vi "LV2013 eZAuto Detect Arduino.vi"(8 "error in (no error)":errorcluster) -> (0 "error out":errorcluster, 2 "Board Type (Uno)":T1, 3 "VISA resource name":refnum<visa-resource-name>)   [LabVIEW 2013]
doc: "Based on the original LIFA base, It returns the Board type as well"
uses:
  <vilib>/LabVIEW Interface for Arduino/Type Defs/Board Type.ctl
  <vilib>/LabVIEW Interface for Arduino/LabVIEW Interface for Arduino.lvlib
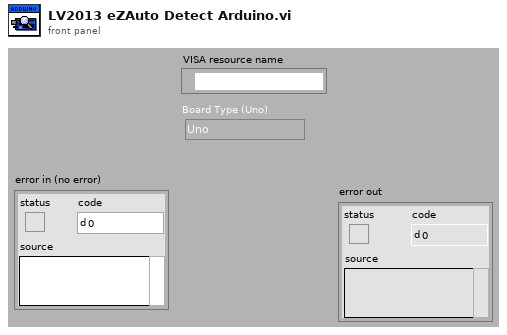
[diagram p1: front panel]
types:
  T1 = typedef "LabVIEW Interface for Arduino.lvlib/Board Type.ctl" = enum16{"Uno", "Dimuelanove w/Atmega 328", "Mega 2560"}
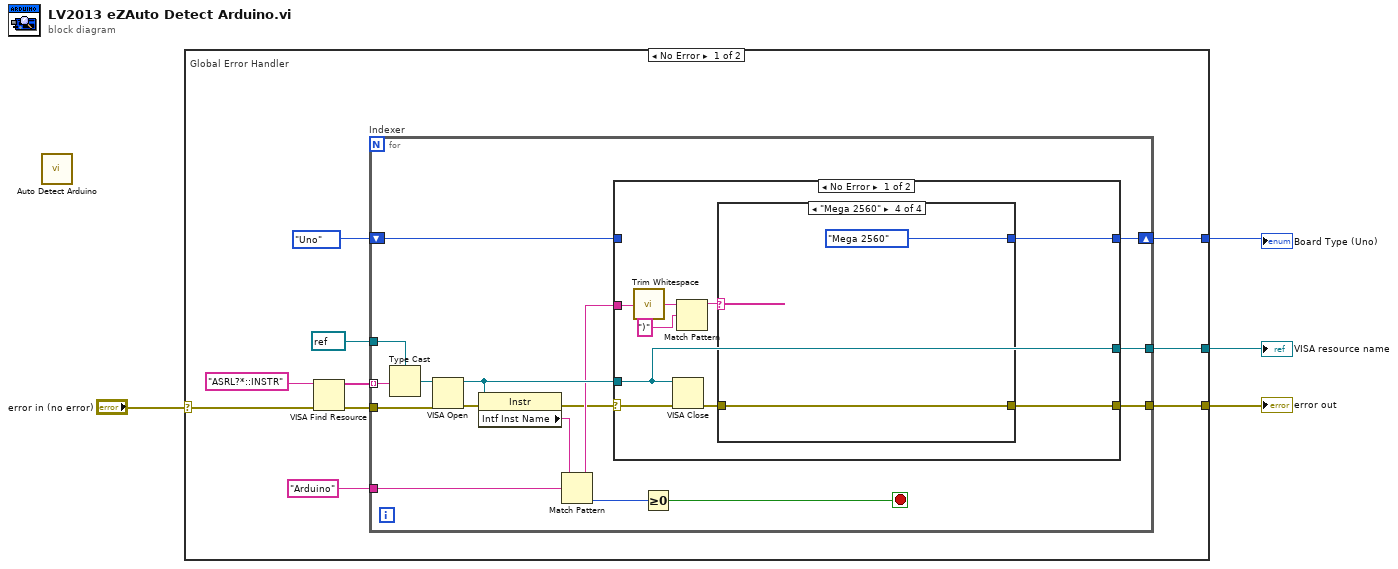
[diagram p0: block diagram]
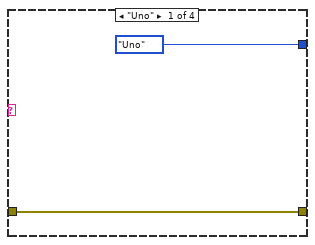
[diagram p2: hidden frame]
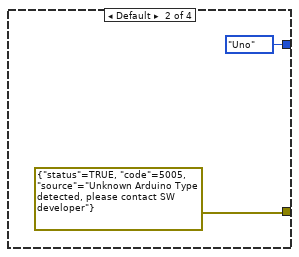
[diagram p3: hidden frame]
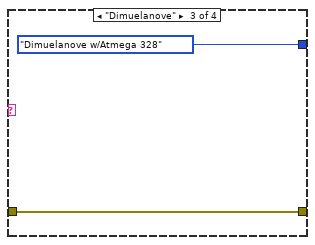
[diagram p4: hidden frame]
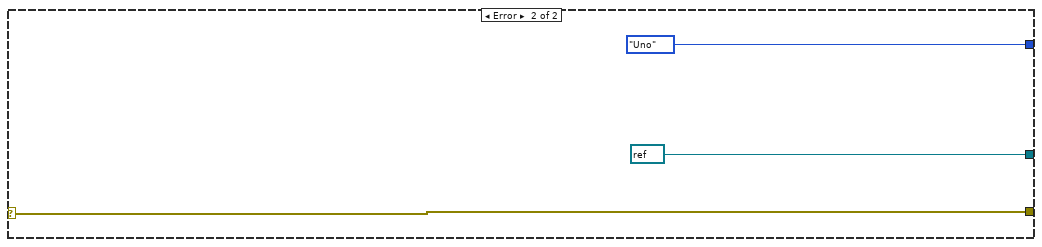
[diagram p6: hidden frame]
diagram:
  n1 = call <vilib>:"Auto Detect Arduino.vi"() -> ()  [unwired: 14 in, 2 out]
  n2 = case "Global Error Handler" shown="No Error" "error in (no error)" {
    selector: "error in (no error)" -> [w9 w51]
    tunnel: [w7 refnum<visa-resource-name> refnum ("VISA resource name")] -> w3
    tunnel: [w10 Board_Type."Uno" ("Board Type (Uno)")] -> w2
    tunnel: [w6 w51] -> w1
    frame No Error {
      n3 = VISA Find Resource(8:w9, 11:"ASRL?*::INSTR" ("expression (\"\")")) -> (0:w8:errorcluster, 3:w13:string[])  [unwired: 1 in, 1 out]
      n4 = for "Indexer" {
        tunnel: w13 -> [w29] mode=indexing
        tunnel: refnum<visa-resource-name> refnum ("VISA resource name") -> [w30]
        shift-right: [w26] -> w10
        shift-left: Board_Type."Uno" ("Board Type (Uno)") -> [w27]
        tunnel: w8 -> [w25]
        tunnel: [w17] -> w7
        tunnel: [w16] -> w6
        tunnel: "Arduino" -> [w15]
        stop <- w18 stop-if-true
        n5 = Type Cast(type=w30, x=w29) -> (*(type *) &x=w28:refnum<visa-resource-name>)
        n6 = VISA Open(error in (no error)=w25, VISA resource name=w28) -> (VISA resource name=w24:refnum<visa-resource-name>, error out=w20:errorcluster)  [unwired: 3 in]
        n7 = property class="Instr"(reference=w24, error in=w20) -> (error out=w19:errorcluster, "Intf Inst Name"=w23:string)  [unwired: 1 out]
        n8 = Match Pattern(string=w23, regular expression=w15) -> (after substring=w21:string, offset past match=w22:i32)  [unwired: 1 in, 2 out]
        n9 = case shown="No Error" w19 {
          selector: w19 -> [w38 w49]
          tunnel: w24 -> [w37 w48]
          tunnel: w27 -> [_ w50]
          tunnel: [w39 w50] -> w26
          tunnel: w21 -> [w36 _]
          tunnel: [w32 w49] -> w16
          tunnel: [w37 w48] -> w17
          frame No Error {
            n10 = call <vilib>:"Trim Whitespace.vi"("string"=w36) -> ("trimmed string"=w35:string)  [unwired: 1 in]
            n11 = VISA Close(VISA resource name=w37, error in (no error)=w38) -> (error out=w31:errorcluster)
            n12 = Match Pattern(string=w35, regular expression=")") -> (before substring=w33:string)  [unwired: 1 in, 3 out]
            n13 = case shown="\"Mega 2560\"" w33 {
              tunnel: [Board_Type."Uno" ("Board Type (Uno)") Board_Type."Uno" ("Board Type (Uno)") Board_Type."Dimuelanove w/Atmega 328" ("Board Type (Uno)") Board_Type."Mega 2560" ("Board Type (Uno)")] -> w39
              tunnel: [w40 errorcluster {"status"=TRUE, "code"=5005, "source"="Unknown Arduino Type detected, please contact SW developer"} ("error out") w44 w46] -> w32
              tunnel: w31 -> [w40 _ w44 w46]
              frame "Uno" {
              }
              frame Default {
              }
              frame "Dimuelanove" {
              }
              frame "Mega 2560" {
              }
            }
          }
          frame Error {
          }
        }
        n14 = Greater Or Equal To 0?(x=w22) -> (x >= 0?=w18:bool)
      }
    }
    frame Error {
    }
  }
  "Board Type (Uno)" <- w2
  "VISA resource name" <- w3
  "error out" <- w1
